vi "备份参数.vi"() -> (0 "仪器公式":T2(array[cluster]), 1 "量程参数":T3(array[cluster]), 2 "试剂容量参数":T4, 3 "外设参数":cluster{"仪器版本":T1, "error out":errorcluster}, 5 "备份结果":string)   [LabVIEW 2016, in "斯坦道CODcr.lvlib"]
uses:
  <vilib>/NI/Progress Bar/Progress Bar.lvlib
  <vilib>/Utility/config.llb/NI_LVConfig.lvlib
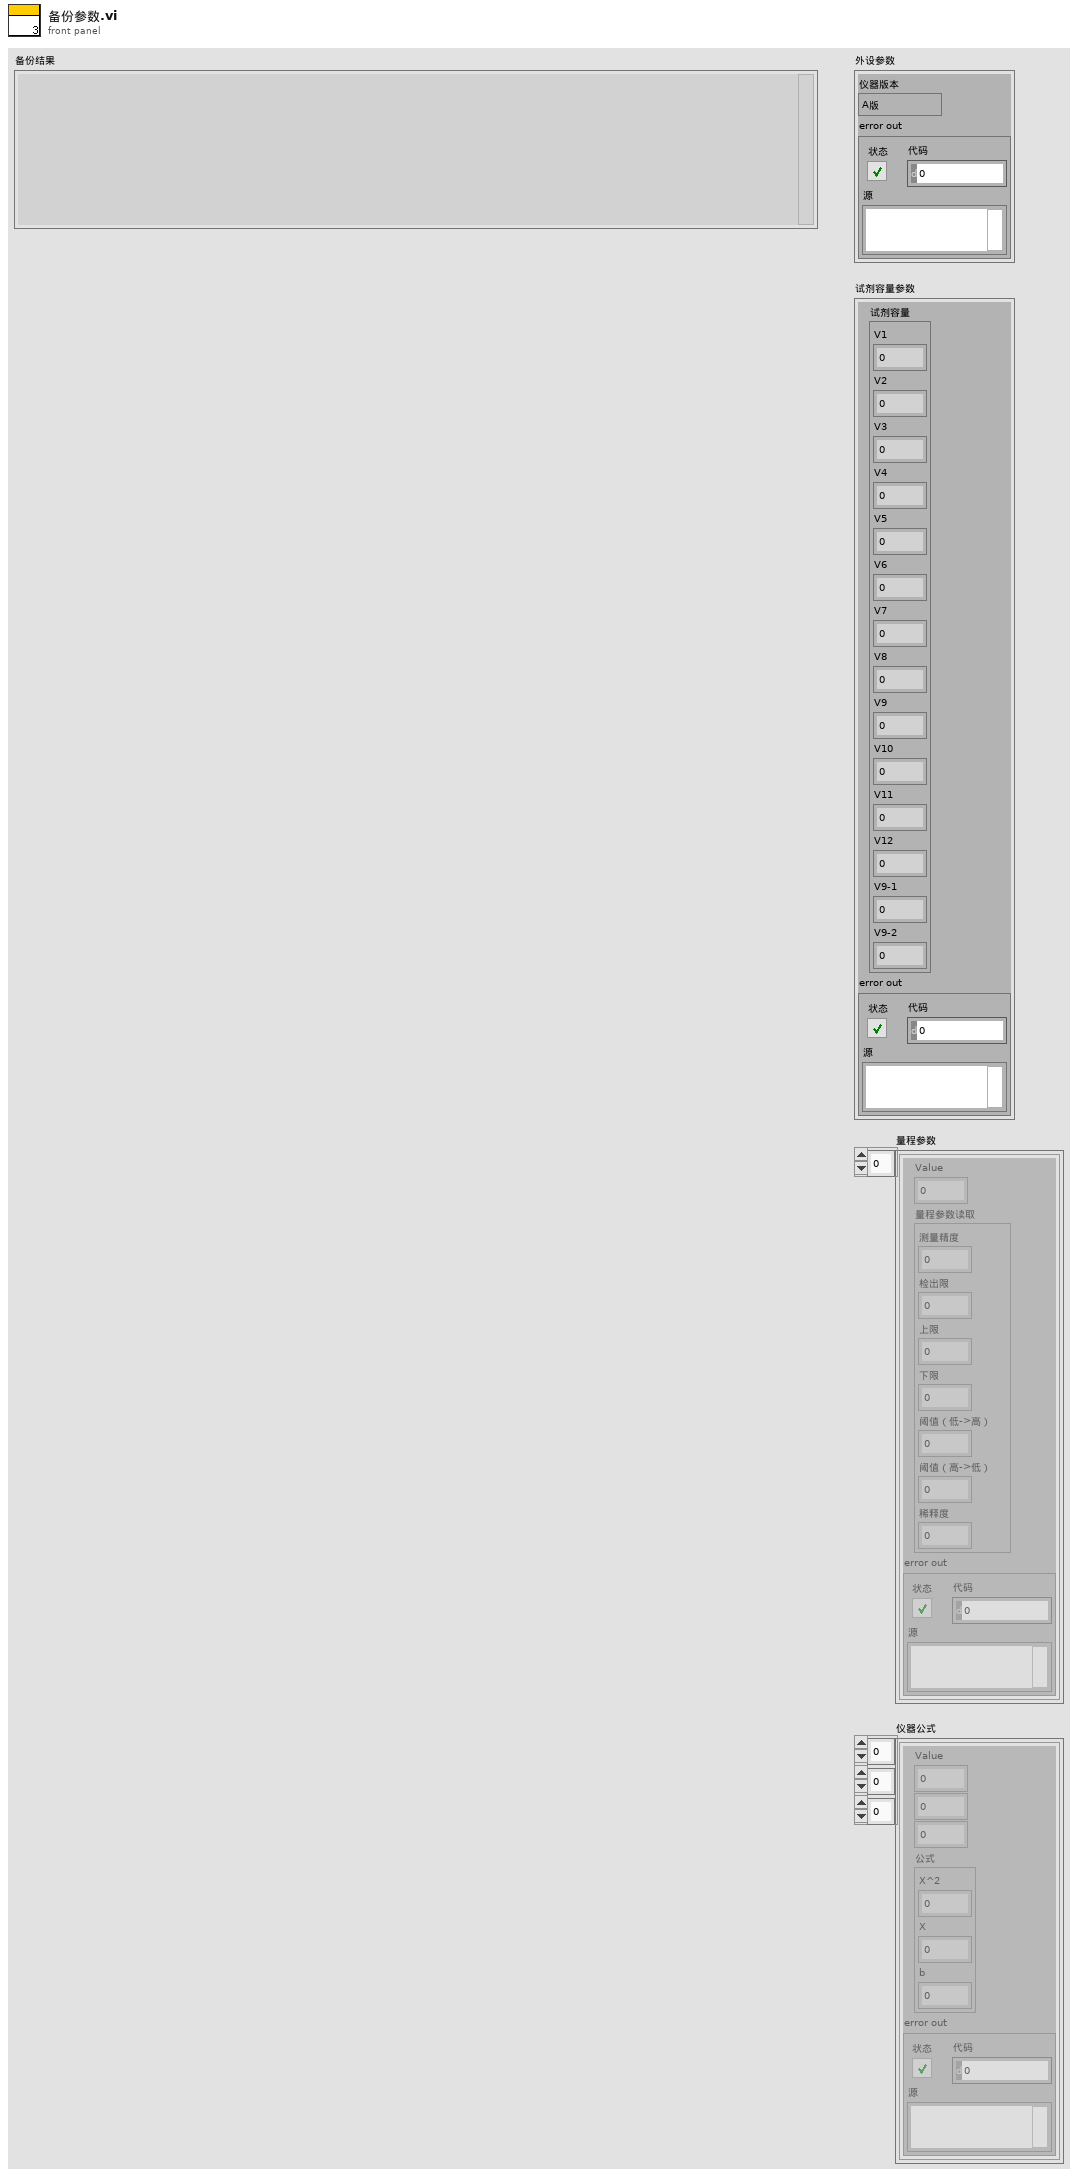
[diagram p1: front panel]
types:
  T1 = typedef "SingleStepTestV3.lvlib/SingleStepTestV3.lvclass/仪器版本.ctl" = enum16{"A版", "B版", "A1版"}
  T2 = cluster{"Value":u16, i32, i32, "公式":cluster{"X^2":dbl, "X":dbl, "b":dbl}, "error out":errorcluster}[][][]
  T3 = cluster{"Value":u16, "量程参数读取":cluster{"测量精度":u16, "检出限":dbl, "上限":dbl, "下限":dbl, "阈值（低->高）":dbl, "阈值（高->低）":dbl, "稀释度":dbl}, "error out":errorcluster}[]
  T4 = cluster{"试剂容量":cluster{"V1":sgl, "V2":sgl, "V3":sgl, "V4":sgl, "V5":sgl, "V6":sgl, "V7":sgl, "V8":sgl, "V9":sgl, "V10":sgl, "V11":sgl, "V12":sgl, "V9-1":sgl, "V9-2":sgl}, "error out":errorcluster}
  T5 = enum16{"备份外设参数", "备份试剂容量参数", "备份量程参数", "备份仪器公式", "结束"}
  T6 = typedef "NI_LVConfig.lvlib/Config Data RefNum.ctl" = refnum<k1>
  T7 = typedef "斯坦道CODcr.lvlib/V3 A版外设参数.ctl" = cluster{"泵类型":u8, "进样速度":u32, "出样速度":u32, "泵阀量":u8, "阀方向":u8, "光谱仪类型":u8, "光谱采样次数":u8, "氙灯次数":u8, "B":u16, "C":u16, "D":u16, "E":u16, "B_COD":u16, "C_COD":u16, "D_COD":u16, "E_COD":u16, "G":u16, "M":u16, "N":u16, "氨氮注射泵控温下限":sgl, "氨氮注射泵控温上限":sgl, "总氮注射泵控温下限":sgl, "总氮注射泵控温上限":sgl, "消解温度下限":sgl, "消解温度上限":sgl, "加热10s限值":sgl, "KP":sgl, "KI":sgl, "KD":sgl, "高温高压阀开阀温度":sgl, "总氮x公式0":u8, "总氮x公式1":sgl, "总氮x公式2":sgl, "总磷浊度稀释系数":sgl, "总磷浊度补偿权重1":sgl, "总磷浊度补偿权重2":sgl, "盐度系数":sgl, "氨氮补偿系数1":sgl, "氨氮补偿系数2":sgl}
  T8 = typedef "斯坦道CODcr.lvlib/V3 B版外设参数.ctl" = cluster{"泵类型":u8, "注射泵正常速度":u32, "注射泵慢速":u32, "阀型号":u8, "res":u8, "光谱仪类型":u8, "光谱采样次数":u8, "氙灯次数":u8, "B":u16, "C":u16, "D":u16, "E":u16, "B_COD":u16, "C_COD":u16, "D_COD":u16, "E_COD":u16, "G":u16, "M":u16, "N":u16, "降温下限":sgl, "降温上限":sgl, "恒温温度下限":sgl, "恒温温度上限":sgl, "消解温度下限":sgl, "消解温度上限":sgl, "加热10s限值":sgl, "KP":sgl, "KI":sgl, "KD":sgl, "高温高压阀开阀温度":sgl, "总氮x公式0":u8, "总氮x公式1":sgl, "总氮x公式2":sgl, "总磷浊度稀释系数":sgl, "总磷浊度补偿权重1":sgl, "总磷浊度补偿权重2":sgl, "盐度系数":sgl, "氨氮补偿系数1":sgl, "氨氮补偿系数2":sgl, "缺试剂传感器阈值":u16}
  T9 = typedef "斯坦道CODcr.lvlib/V3 A1版外设参数.ctl" = cluster{"泵类型":u8, "进样速度":u32, "出样速度":u32, "泵阀量":u8, "光谱仪类型":u8, "光谱采样次数":u8, "氙灯次数":u8, "B":u16, "C":u16, "D":u16, "E":u16, "B_COD":u16, "C_COD":u16, "D_COD":u16, "E_COD":u16, "G":u16, "M":u16, "N":u16, "氨氮注射泵控温下限":sgl, "氨氮注射泵控温上限":sgl, "总氮注射泵控温下限":sgl, "总氮注射泵控温上限":sgl, "消解温度下限":sgl, "消解温度上限":sgl, "加热10s限值":sgl, "高温高压阀开阀温度":sgl, "总氮x公式0":u8, "总氮x公式1":sgl, "总氮x公式2":sgl, "总磷浊度稀释系数":sgl, "总磷浊度补偿权重1":sgl, "总磷浊度补偿权重2":sgl, "盐度系数":sgl, "氨氮补偿系数1":sgl, "氨氮补偿系数2":sgl}
  T10 = cluster{"V1":sgl, "V2":sgl, "V3":sgl, "V4":sgl, "V5":sgl, "V6":sgl, "V7":sgl, "V8":sgl, "V9":sgl, "V10":sgl, "V11":sgl, "V12":sgl, "V9-1":sgl, "V9-2":sgl}
  T11 = cluster{"测量精度":u16, "检出限":dbl, "上限":dbl, "下限":dbl, "阈值（低->高）":dbl, "阈值（高->低）":dbl, "稀释度":dbl}
  T12 = cluster{"Value":u16, "量程参数读取":cluster{"测量精度":u16, "检出限":dbl, "上限":dbl, "下限":dbl, "阈值（低->高）":dbl, "阈值（高->低）":dbl, "稀释度":dbl}, "error out":errorcluster}
  T13 = cluster{"Value":u16, i32, i32, "公式":cluster{"X^2":dbl, "X":dbl, "b":dbl}, "error out":errorcluster}
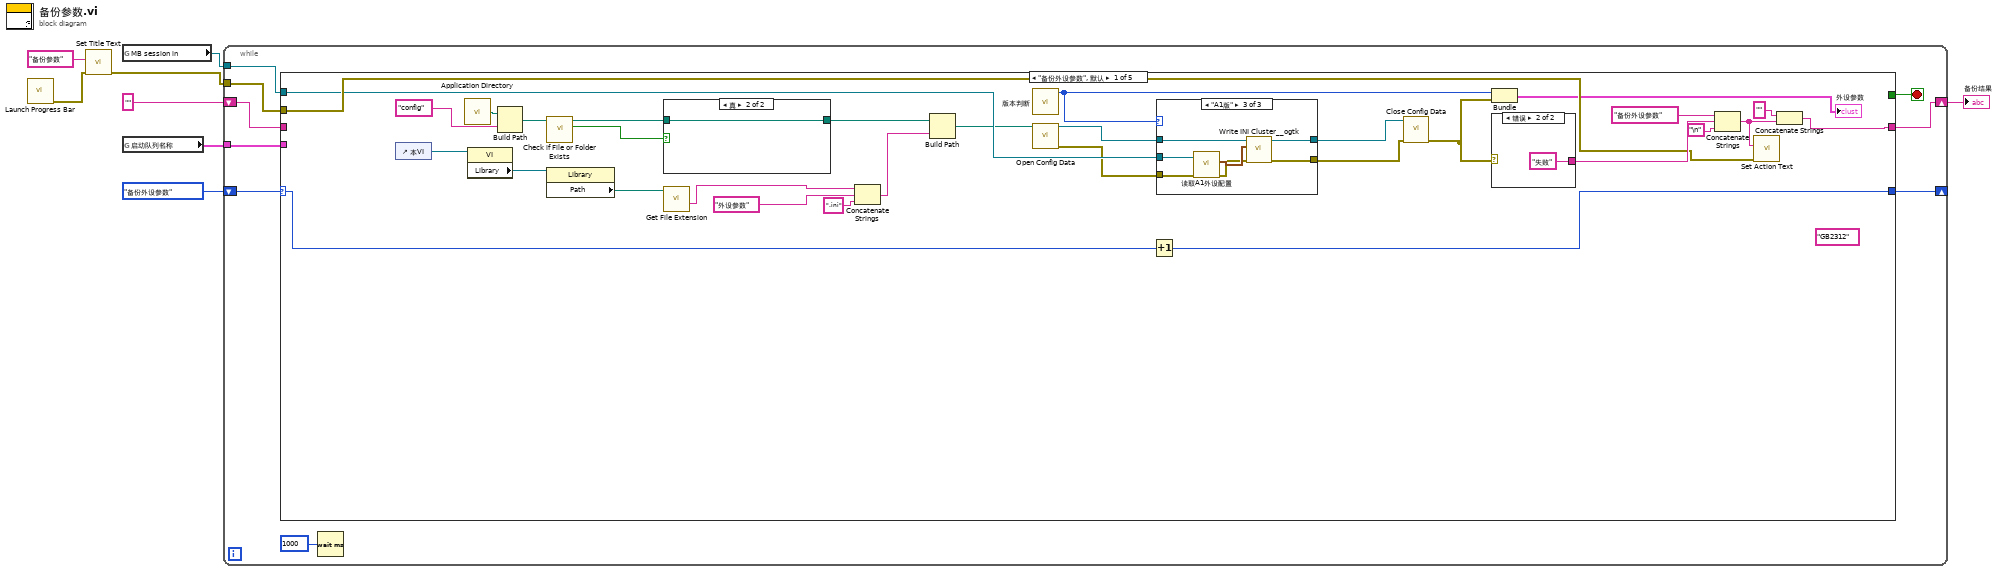
[diagram p0: block diagram]
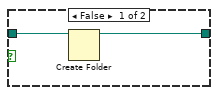
[diagram p2: hidden frame]
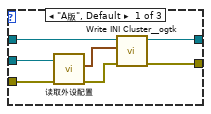
[diagram p3: hidden frame]
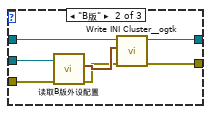
[diagram p4: hidden frame]
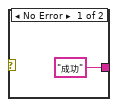
[diagram p5: hidden frame]
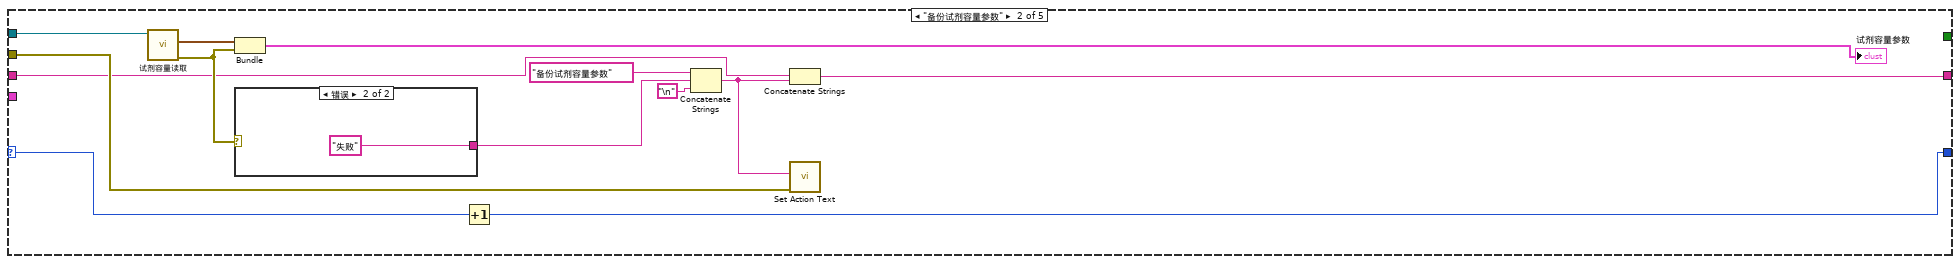
[diagram p6: hidden frame]
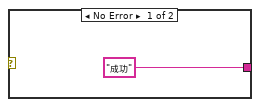
[diagram p7: hidden frame]
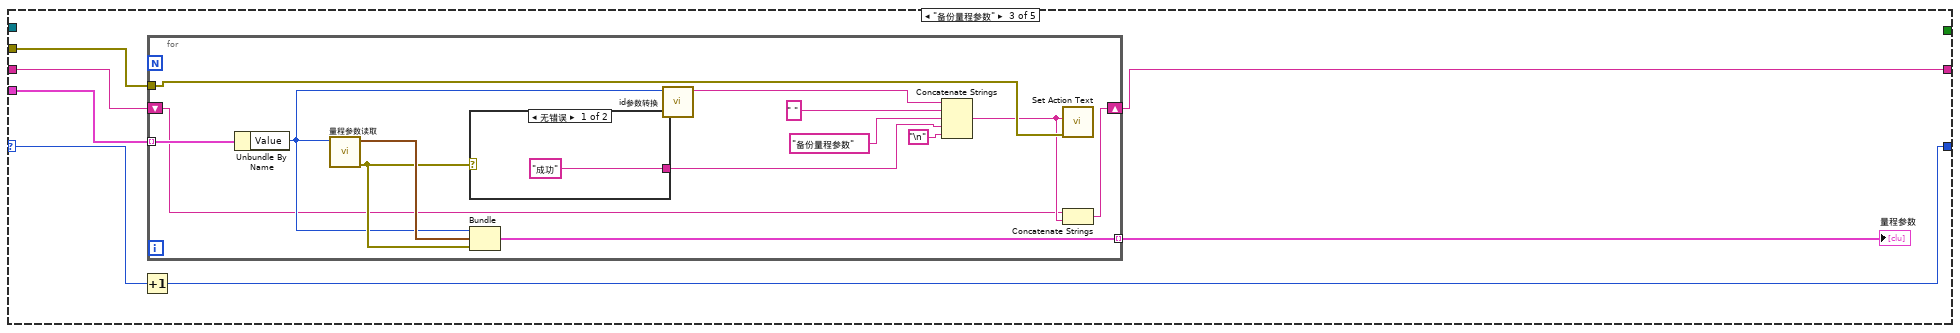
[diagram p8: hidden frame]
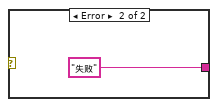
[diagram p9: hidden frame]
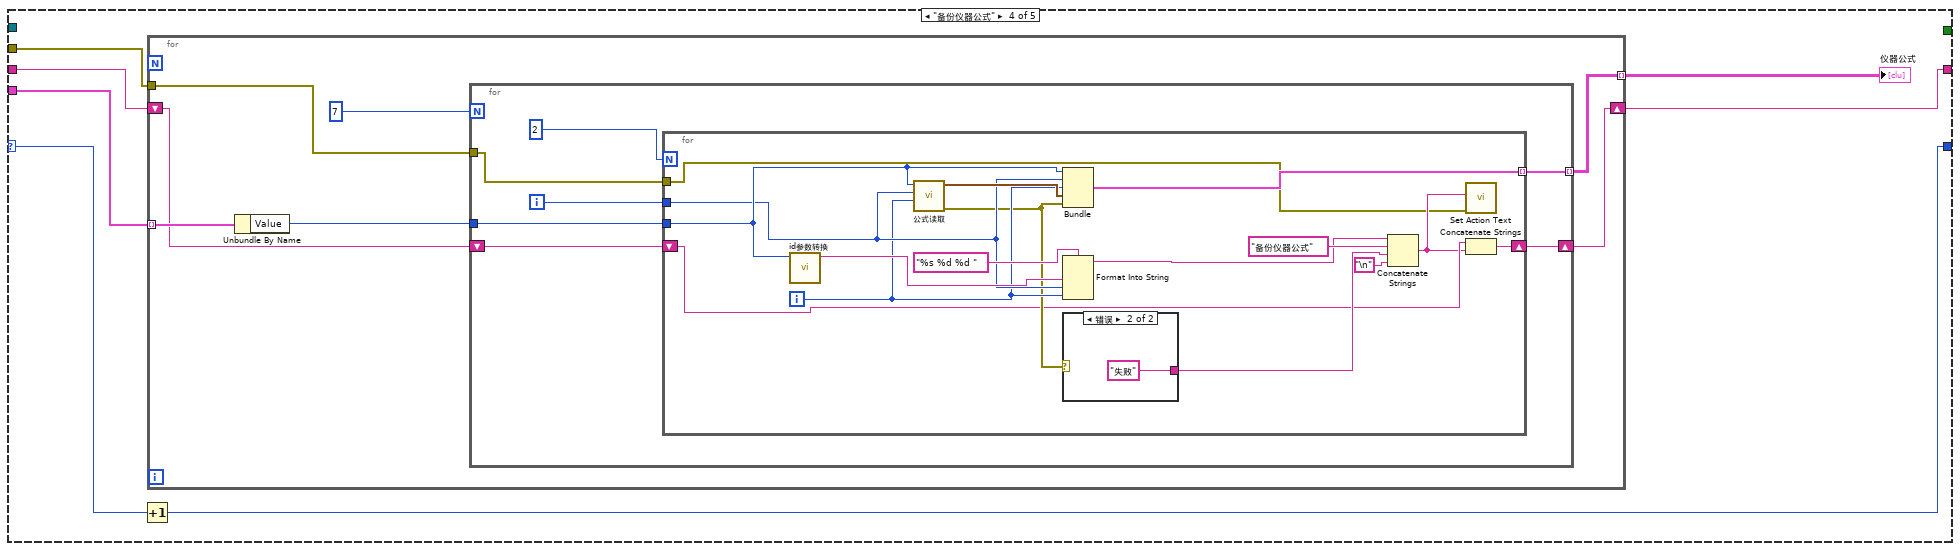
[diagram p10: hidden frame]
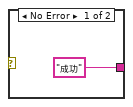
[diagram p11: hidden frame]
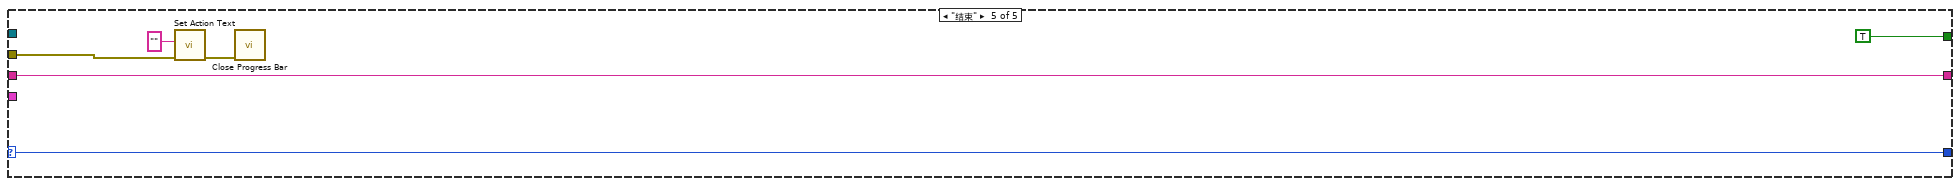
[diagram p12: hidden frame]
diagram:
  n1 = call <vilib>:"Launch Progress Bar.vi"() -> ("error out"=w3:errorcluster)  [unwired: 10 in, 1 out]
  n2 = call <vilib>:"Set Title Text.vi"("error in (no error)"=w3, "Installer Title"="备份参数") -> ("error out"=w2:errorcluster)  [unwired: 9 in]
  n3 = global read "VAR总磷总氮全局变量.vi" "MB session in"() -> (w7:refnum<class "MB_Master.lvclass">)
  n4 = global read "model config var.vi" "启动队列名称"() -> (w5:cluster{"String":string, "Value":u16}[])
  n5 = while {
    shift-right: [w13] -> _
    shift-left: T5."备份外设参数" ("枚举") -> [w16]
    tunnel: w7 -> [w17]
    shift-right: [w14] -> w4
    shift-left: "" -> [w15]
    tunnel: w5 -> [w12]
    tunnel: w2 -> [w10]
    stop <- w11 stop-if-true
    n6 = case shown="\"备份外设参数\", 默认" w16 {
      selector: w16 -> [w45 w81 w93 w116 w157]
      tunnel: w17 -> [w39 w87 _ _ _]
      tunnel: w15 -> [_ w77 w95 w118 w156]
      tunnel: [w42 w75 w94 w117 w156] -> w14
      tunnel: [w44 w80 w92 w115 w157] -> w13
      tunnel: w12 -> [_ _ w96 w119 _]
      tunnel: [_ _ _ _ TRUE] -> w11
      tunnel: w10 -> [w40 w78 w90 w113 w154]
      frame "备份外设参数", Default {
        (unwired) "GB2312" ("XML Encoding")
        n7 = control-ref of="本VI"() -> (w25:refnum<vi>)
        n8 = call <vilib>:"Application Directory.vi"() -> ("Application Directory"=w35:path)
        n9 = property class="VI"(reference=w25) -> ("Library"=w37:refnum<vi>)  [unwired: 1 in, 2 out]
        n10 = Build Path(base path=w35, name or relative path="config" ("名称或相对路径")) -> (appended path=w33:path)
        n11 = call <vilib>:"Check if File or Folder Exists.vi"("path"=w33) -> ("file or folder exists?"=w30:bool, "dup path"=w29:path)  [unwired: 8 in, 1 out]
        n12 = property class="Library"(reference=w37) -> ("Path"=w36:path)  [unwired: 1 in, 2 out]
        n13 = case shown="真" w30 {
          tunnel: w29 -> [w50 w51]
          tunnel: [w49 w51] -> w28
          frame False {
            n14 = Create Folder(path (use dialog)=w50) -> (created path=w49:path)  [unwired: 2 in, 2 out]
          }
          frame True {
          }
        }
        n15 = call <vilib>:"Get File Extension.vi"("file"=w36) -> ("filename without extension"=w27:string)  [unwired: 6 in, 4 out]
        n16 = Concatenate Strings(w27, "外设参数" ("字符串"), ".ini" ("字符串")) -> (w31:string)
        n17 = Build Path(base path=w28, name or relative path=w31) -> (appended path=w23:path)
        n18 = call "版本判断.vi"() -> ("仪器版本"=w24:T1)  [unwired: 11 in]
        n19 = call <vilib>:"Open Config Data.vi"("configuration file path"=w23) -> ("error out"=w20:errorcluster, "refnum"=w22:T6)  [unwired: 8 in, 1 out]
        n20 = Increment(x=w45) -> (x+1=w44:T5)
        n21 = case shown="\"A1版\"" w24 {
          tunnel: [w52 w59 w66] -> w19
          tunnel: w39 -> [w58 w65 w72]
          tunnel: w22 -> [w54 w64 w71]
          tunnel: [w53 w62 w69] -> w21
          tunnel: w20 -> [w57 w61 w68]
          frame "A版", Default {
            n22 = call "读取外设配置.vi"("error in (no error)"=w57, "MB session in"=w58) -> ("error out"=w56:errorcluster, "外设配置"=w55:T7)  [unwired: 7 in, 1 out]
            n23 = call <userlib>:"Write INI Cluster__ogtk.vi"("error in (no error)"=w56, "INI Fomatted Cluster"=w55, "refnum"=w54) -> ("error out"=w52:errorcluster, "dup refnum"=w53:T6)  [unwired: 7 in]
          }
          frame "B版" {
            n24 = call "读取B版外设配置.vi"("error in (no error)"=w61, "MB session in"=w65) -> ("error out"=w60:errorcluster, "外设配置"=w63:T8)  [unwired: 7 in, 1 out]
            n25 = call <userlib>:"Write INI Cluster__ogtk.vi"("error in (no error)"=w60, "INI Fomatted Cluster"=w63, "refnum"=w64) -> ("error out"=w59:errorcluster, "dup refnum"=w62:T6)  [unwired: 7 in]
          }
          frame "A1版" {
            n26 = call "读取A1外设配置.vi"("error in (no error)"=w68, "MB session in"=w72) -> ("error out"=w67:errorcluster, "外设配置"=w70:T9)  [unwired: 7 in, 1 out]
            n27 = call <userlib>:"Write INI Cluster__ogtk.vi"("error in (no error)"=w67, "INI Fomatted Cluster"=w70, "refnum"=w71) -> ("error out"=w66:errorcluster, "dup refnum"=w69:T6)  [unwired: 7 in]
          }
        }
        n28 = call <vilib>:"Close Config Data.vi"("error in (no error)"=w19, "refnum"=w21) -> ("error out"=w18:errorcluster)  [unwired: 8 in, 1 out]
        n29 = Bundle("仪器版本"=w24, "error out"=w18) -> (→"外设参数":cluster{"仪器版本":T1, "error out":errorcluster})  [unwired: 1 in]
        n30 = case shown="错误" w18 {
          tunnel: ["成功" "失败"] -> w48
          frame No Error {
          }
          frame Error {
          }
        }
        n31 = Concatenate Strings("备份外设参数" ("字符串"), w48, "\n") -> (w43:string)
        n32 = call <vilib>:"Set Action Text.vi"("error in (no error)"=w40, "Action Text"=w43) -> ()  [unwired: 9 in, 1 out]
        n33 = Concatenate Strings("" ("字符串"), w43) -> (w42:string)
      }
      frame "备份试剂容量参数" {
        n34 = call "试剂容量读取.vi"("MB session in"=w87) -> ("error out"=w82:errorcluster, "试剂容量"=w86:T10)  [unwired: 8 in, 1 out]
        n35 = Bundle("试剂容量"=w86, "error out"=w82) -> (→"试剂容量参数":T4)  [unwired: 1 in]
        n36 = case shown="错误" w82 {
          tunnel: ["成功" "失败"] -> w85
          frame No Error {
          }
          frame Error {
          }
        }
        n37 = Increment(x=w81) -> (x+1=w80:T5)
        n38 = Concatenate Strings("备份试剂容量参数" ("字符串"), w85, "\n") -> (w76:string)
        n39 = Concatenate Strings(w77, w76) -> (w75:string)
        n40 = call <vilib>:"Set Action Text.vi"("error in (no error)"=w78, "Action Text"=w76) -> ()  [unwired: 9 in, 1 out]
      }
      frame "备份量程参数" {
        n41 = Increment(x=w93) -> (x+1=w92:T5)
        n42 = for {
          tunnel: w96 -> [w110] mode=indexing
          tunnel: [w108] -> w91 mode=indexing
          shift-right: [w97] -> w94
          shift-left: w95 -> [w98]
          tunnel: w90 -> [w100]
          n43 = Unbundle By Name(w110) -> ("Value"=w104:u16)
          n44 = call "量程参数读取.vi"("测量参数"=w104) -> ("error out"=w105:errorcluster, "量程参数读取"=w109:T11)  [unwired: 9 in]
          n45 = case shown="无错误" w105 {
            tunnel: ["成功" "失败"] -> w107
            frame No Error {
            }
            frame Error {
            }
          }
          n46 = Bundle("Value"=w104, "量程参数读取"=w109, "error out"=w105) -> (w108:T12)  [unwired: 1 in]
          n47 = call "id参数转换.vi"("id"=w104) -> ("table输出"=w103:string)  [unwired: 9 in, 1 out]
          n48 = Concatenate Strings(w103, " " ("字符串"), "备份量程参数" ("字符串"), w107, "\n") -> (w99:string)
          n49 = call <vilib>:"Set Action Text.vi"("error in (no error)"=w100, "Action Text"=w99) -> ()  [unwired: 9 in, 1 out]
          n50 = Concatenate Strings(w98, w99) -> (w97:string)
        }
        "量程参数" <- w91
      }
      frame "备份仪器公式" {
        n51 = Increment(x=w116) -> (x+1=w115:T5)
        n52 = for {
          tunnel: w119 -> [w126] mode=indexing
          tunnel: [w123] -> w114 mode=indexing
          shift-right: [w121] -> w117
          shift-left: w118 -> [w122]
          tunnel: w113 -> [w120]
          n53 = Unbundle By Name(w126) -> ("Value"=w124:u16)
          n54 = for {
            N: 7 -> [_]
            tunnel: w124 -> [w133]
            tunnel: [w130] -> w123 mode=indexing
            shift-right: [w129] -> w121
            shift-left: w122 -> [w128]
            tunnel: w120 -> [w127]
            i -> [w132]
            n55 = for {
              N: 2 -> [_]
              tunnel: w133 -> [w145]
              tunnel: w132 -> [w142]
              tunnel: [w148] -> w130 mode=indexing
              shift-right: [w134] -> w129
              shift-left: w128 -> [w137]
              tunnel: w127 -> [w135]
              i -> [w141]
              n56 = call "id参数转换.vi"("id"=w145) -> ("table输出"=w143:string)  [unwired: 9 in, 1 out]
              n57 = call "公式读取.vi"("量程"=w141, "测量模式"=w142, "测量参数"=w145) -> ("error out"=w139:errorcluster, "公式"=w149:cluster{"X^2":dbl, "X":dbl, "b":dbl})  [unwired: 7 in]
              n58 = Bundle("Value"=w145, w142, w141, "公式"=w149, "error out"=w139) -> (w148:T13)  [unwired: 1 in]
              n59 = Format Into String(format string="%s %d %d " ("格式字符串"), w143, w142, w141) -> (resulting string=w140:string)  [unwired: 2 in, 1 out]
              n60 = case shown="错误" w139 {
                tunnel: ["成功" "失败"] -> w147
                frame No Error {
                }
                frame Error {
                }
              }
              n61 = Concatenate Strings(w140, "备份仪器公式" ("字符串"), w147, "\n") -> (w136:string)
              n62 = call <vilib>:"Set Action Text.vi"("error in (no error)"=w135, "Action Text"=w136) -> ()  [unwired: 9 in, 1 out]
              n63 = Concatenate Strings(w137, w136) -> (w134:string)
            }
          }
        }
        "仪器公式" <- w114
      }
      frame "结束" {
        n64 = call <vilib>:"Set Action Text.vi"("error in (no error)"=w154, "Action Text"="") -> ("error out"=w152:errorcluster)  [unwired: 9 in]
        n65 = call <vilib>:"Close Progress Bar.vi"("error in (no error)"=w152) -> ()  [unwired: 9 in, 2 out]
      }
    }
    n66 = Wait (ms)(milliseconds to wait=u32 1000 ("等待时间（毫秒）")) -> ()  [unwired: 1 out]
  }
  "备份结果" <- w4
